vi "Write Data To Queue.vi"(8 "error in (no error)":errorcluster, 11 "StateAuto in":refnum<class "StateAuto.lvclass">) -> (0 "error out":errorcluster, 3 "StateAuto out":refnum<class "StateAuto.lvclass">)   [LabVIEW 2017, in "LibraryGcode.lvlib" / "StateAuto.lvclass"]
uses:
  StateAuto.lvclass
  StateAuto.lvclass/StateAuto.ctl
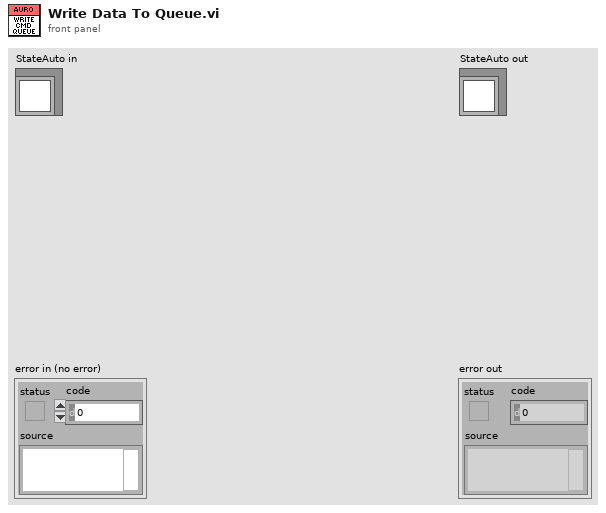
[diagram p1: front panel]
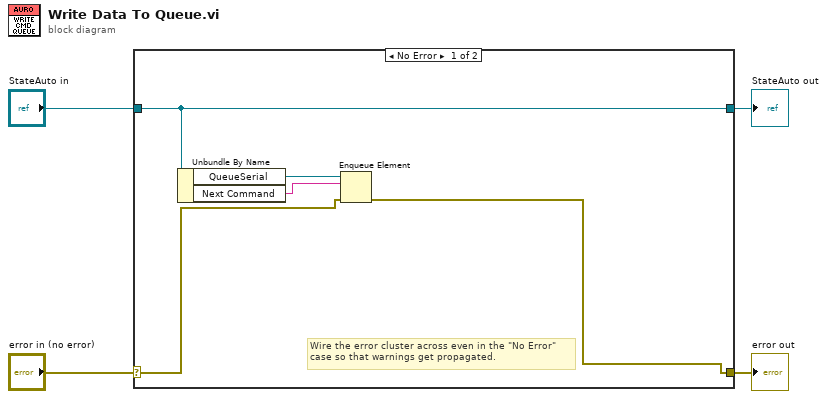
[diagram p0: block diagram]
diagram:
  n1 = case shown="No Error" "error in (no error)" {
    selector: "error in (no error)" -> [w6 w11]
    tunnel: [w5 w11] -> w3
    tunnel: [w9 w10] -> w1
    tunnel: "StateAuto in" -> [w9 w10]
    frame No Error {
      # "Wire the error cluster across even in the \"No Error\"\ncase so that warnings get propagated."
      n2 = Unbundle By Name(w9) -> ("QueueSerial"=w8:refnum<queue>, "Next Command"=w7:string)
      n3 = Enqueue Element(queue=w8, element=w7, error in (no error)=w6) -> (error out=w5:errorcluster)  [unwired: 1 in, 2 out]
    }
    frame Error {
    }
  }
  "error out" <- w3
  "StateAuto out" <- w1
